vi "DB_Withdrawal.vi"() -> ()   [LabVIEW 2013, in "ConfigDBLib.lvlib"]
uses:
  ConfigDBLib.lvlib
panel:
  out "Insufficient Fund":bool
  in  "Withdrawal Amount":dbl
  in  "Total Balance":dbl
  in  "Account Number":dbl
  out "error out":errorcluster
  in  "error in (no error)":errorcluster
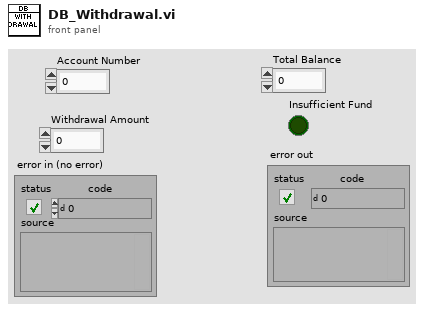
[diagram p1: front panel]
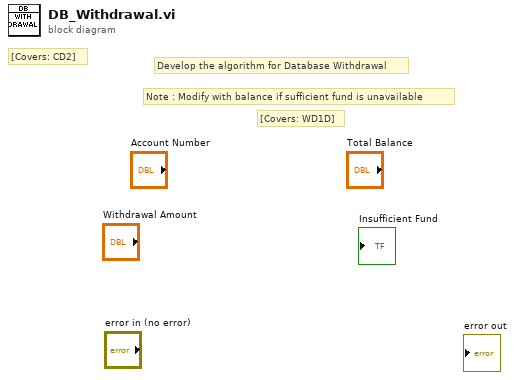
[diagram p0: block diagram]
diagram:
  # "[Covers: WD1D]"
  # "Note : Modify with balance if sufficient fund is unavailable"
  # "[Covers: CD2]"
  # "Develop the algorithm for Database Withdrawal"
